vi "Send M.vi"(8 "error in (no error)":errorcluster, 11 "H3611i Actor in":refnum<class "H3611i Actor.lvclass">) -> (0 "error out":errorcluster, 3 "H3611i Actor out":refnum<class "H3611i Actor.lvclass">)   [LabVIEW 2018, in "H3611i.lvlib" / "H3611i Actor.lvclass"]
uses:
  H3611i Actor.lvclass
  C:/Users/dev/Documents/CODE/LabVIEW/microwaveverify/trunk/MWWL Verification/Sensor Actor/Sensor/Sensor.lvclass
  H3611i Actor.lvclass/H3611i Actor.ctl
  Sensor Actor/Sensor/Sensor.lvclass
panel:
  in  "milliseconds to wait":u32=500
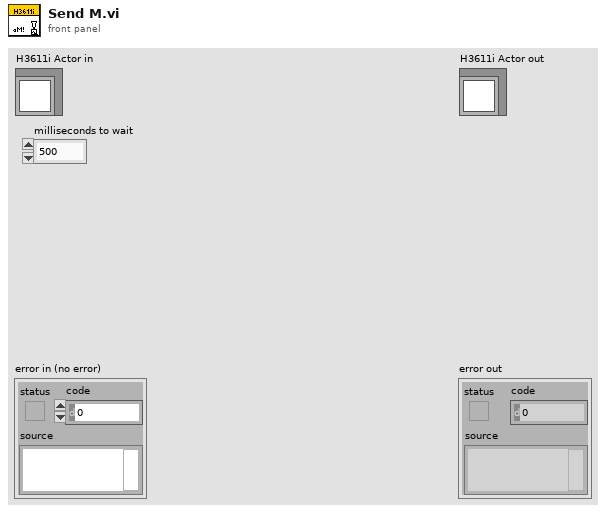
[diagram p1: front panel]
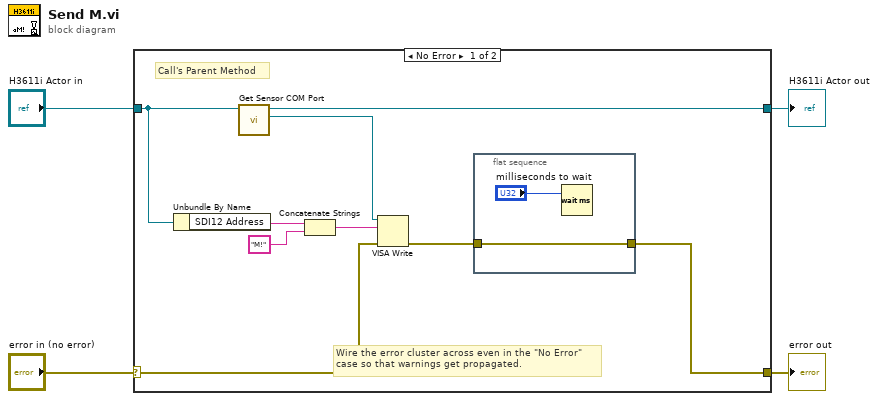
[diagram p0: block diagram]
diagram:
  n1 = case shown="No Error" "error in (no error)" {
    selector: "error in (no error)" -> [w7 w17]
    tunnel: [w5 w17] -> w3
    tunnel: [w12 w16] -> w1
    tunnel: "H3611i Actor in" -> [w13 w16]
    frame No Error {
      # "Call's Parent Method"
      # "Wire the error cluster across even in the \"No Error\"\ncase so that warnings get propagated."
      n2 = Unbundle By Name(w13) -> ("SDI12 Address"=w10:string)
      n3 = call "Get Sensor COM Port.vi"("Sensor in"=w13) -> ("COM Port"=w11:refnum<visa-resource-name>, "Sensor out"=w12:refnum<class "H3611i Actor.lvclass">)  [unwired: 8 in, 1 out]
      n4 = Concatenate Strings(w10, "M!" ("string")) -> (w8:string)
      n5 = VISA Write(VISA resource name=w11, write buffer=w8, error in (no error)=w7) -> (error out=w6:errorcluster)  [unwired: 2 out]
      n6 = flat-sequence {
        tunnel: w6 -> [w14]
        tunnel: [w14] -> w5
        frame #0 {
          n7 = Wait (ms)(milliseconds to wait="milliseconds to wait") -> ()  [unwired: 1 out]
        }
      }
    }
    frame Error {
    }
  }
  "error out" <- w3
  "H3611i Actor out" <- w1
